vi "createCellStyle.vi"(8 "error in (no error)":errorcluster, 10 "Style":refnum<class "Style.lvclass">, 11 "MS-Excel in":refnum<class "MS-Excel.lvclass">) -> (0 "error out":errorcluster, 2 "Cell Style":refnum<k24>, 3 "MS-Excel out":refnum<class "MS-Excel.lvclass">)   [LabVIEW 2017, in "LabVIEW NPOI.lvlib" / "MS-Excel.lvclass"]
uses:
  MS-Excel.lvclass
  Styles/Style/Style.lvclass
  C:/Program Files (x86)/National Instruments/LabVIEW 2017/vi.lib/BenjaminR/LabVIEW NPOI/lib/NPOI 2.1.1/NPOI.dll
  Program Files (x86)/National Instruments/LabVIEW 2017/vi.lib/BenjaminR/LabVIEW NPOI/lib/NPOI 2.1.1/NPOI.dll
  MS-Excel.lvclass/MS-Excel.ctl
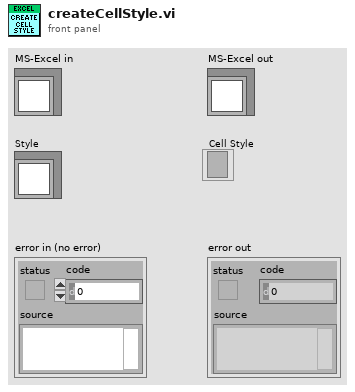
[diagram p1: front panel]
types:
  T1 = typedef "Styles.lvlib/Underline--ring.ctl" = i32
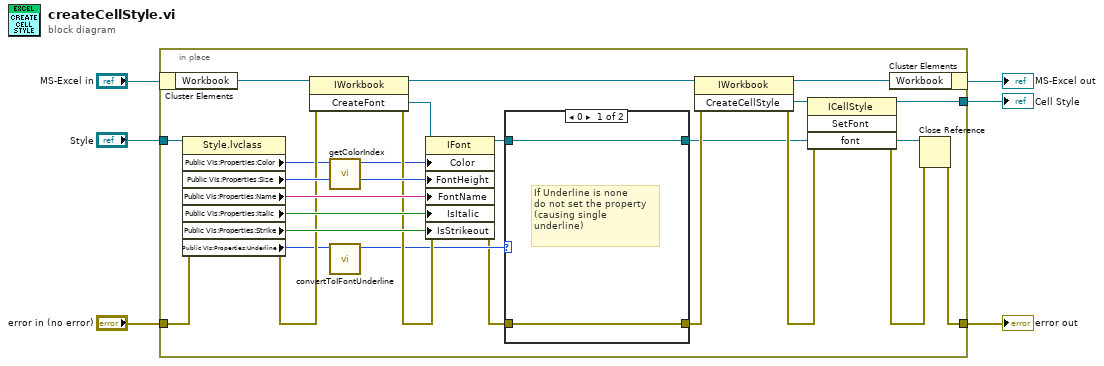
[diagram p0: block diagram]
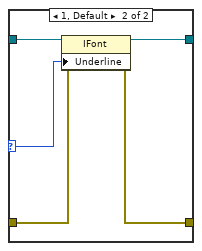
[diagram p2: hidden frame]
diagram:
  n1 = in-place {
    in-place-border: [w19] -> w3
    in-place-border: "error in (no error)" -> [w17]
    in-place-border: "Style" -> [w16]
    in-place-border: [w15] -> w1
    n2 = in-place-cluster #1("MS-Excel in") -> ("Workbook"=w22:refnum<k24>)
    n3 = property class="Style.lvclass"(reference=w16, error in=w17) -> (error out=w18:errorcluster, "Public VIs:Properties:Color"=w13:u32, "Public VIs:Properties:Size"=w27:i32, "Public VIs:Properties:Name"=w28:string, "Public VIs:Properties:Italic"=w29:bool, "Public VIs:Properties:Strike"=w30:bool, "Public VIs:Properties:Underline"=w14:T1)  [unwired: 1 out]
    n4 = invoke class="IWorkbook" method="CreateFont"(reference=w22, error in=w18) -> (reference out=w23:refnum<k24>, error out=w25:errorcluster, "CreateFont"=w26:refnum<k24>)  [unwired: 1 in]
    n5 = call "getColorIndex.vi"("Color"=w13) -> ("excel color table index"=w12:i16)  [unwired: 10 in]
    n6 = call "convertToIFontUnderline.vi"("Underline"=w14) -> ("IFont.Underline"=w11:u8)  [unwired: 10 in]
    n7 = property class="IFont"(reference=w26, error in=w25, "Color"=w12, "FontHeight"=w27, "FontName"=w28, "IsItalic"=w29, "IsStrikeout"=w30) -> (reference out=w8:refnum<k24>, error out=w10:errorcluster)
    n8 = case shown="0" w11 {
      selector: w11 -> [_ w34]
      tunnel: w10 -> [w32 w36]
      tunnel: [w32 w35] -> w9
      tunnel: w8 -> [w33 w38]
      tunnel: [w33 w37] -> w7
      frame 0 {
        # "If Underline is none \ndo not set the property \n(causing single\nunderline)"
      }
      frame 1, Default {
        n9 = property class="IFont"(reference=w38, error in=w36, "Underline"=w34) -> (reference out=w37:refnum<k24>, error out=w35:errorcluster)
      }
    }
    n10 = invoke class="IWorkbook" method="CreateCellStyle"(reference=w23, error in=w9) -> (reference out=w21:refnum<k24>, error out=w31:errorcluster, "CreateCellStyle"=w24:refnum<k24>)  [unwired: 1 in]
    n11 = invoke class="ICellStyle" method="SetFont"(reference=w24, error in=w31, "font"=w7) -> (reference out=w15:refnum<k24>, error out=w20:errorcluster)  [unwired: 1 in, 2 out]
    n12 = in-place-cluster #1("Workbook"=w21) -> (→"MS-Excel out":refnum<class "MS-Excel.lvclass">)
    n13 = Close Reference(reference=w7, error in (no error)=w20) -> (error out=w19:errorcluster)
  }
  "error out" <- w3
  "Cell Style" <- w1
